vi "试验授权.vi"() -> ()   [LabVIEW 2016]
panel:
  out "簇":T1
  in  "R3加载时间/S  4":dbl=30.0
  in  "R2加载时间/S  4":dbl=30.0
  in  "R1加载时间/S  4":dbl=30.0
  in  "D6加载时间/S  4":dbl=30.0
  in  "D5加载时间/S  4":dbl=30.0
  in  "D4加载时间/S  4":dbl=30.0
  in  "D3加载时间/S 4":dbl=30.0
  in  "D2加载时间/S  4":dbl=30.0
  in  "D1加载时间/S 4":dbl=30.0
  in  "R3加载时间/S  3":dbl=30.0
  in  "R2加载时间/S  3":dbl=30.0
  in  "R1加载时间/S  3":dbl=30.0
  in  "D6加载时间/S  3":dbl=30.0
  in  "D5加载时间/S  3":dbl=30.0
  in  "D4加载时间/S  3":dbl=30.0
  in  "D3加载时间/S 3":dbl=30.0
  in  "D2加载时间/S  3":dbl=30.0
  in  "D1加载时间/S 3":dbl=30.0
  in  "R3加载时间/S  2":dbl=30.0
  in  "R2加载时间/S  2":dbl=30.0
  in  "R1加载时间/S  2":dbl=30.0
  in  "D6加载时间/S  2":dbl=30.0
  in  "D5加载时间/S  2":dbl=30.0
  in  "D4加载时间/S  2":dbl=30.0
  in  "D3加载时间/S 2":dbl=30.0
  in  "D2加载时间/S  2":dbl=30.0
  in  "D1加载时间/S 2":dbl=30.0
  in  "SG18-3百分比":dbl min=0.0 max=100.0 step=1.0
  in  "SG16-3百分比":dbl min=0.0 max=100.0 step=1.0
  in  "SG14百分比":dbl min=0.0 max=100.0 step=1.0
  in  "R3加载时间/S":dbl=30.0
  in  "R2加载时间/S":dbl=30.0
  in  "R1加载时间/S":dbl=30.0
  in  "D6加载时间/S":dbl=30.0
  in  "D5加载时间/S":dbl=30.0
  in  "D4加载时间/S":dbl=30.0
  in  "D3加载时间/S":dbl=30.0
  in  "D2加载时间/S":dbl=30.0
  in  "D1加载时间/S":dbl=30.0
  in  "R3":dbl min=0.0 max=100.0 step=1.0
  in  "R2":dbl min=0.0 max=100.0 step=1.0
  in  "R1":dbl min=0.0 max=100.0 step=1.0
  in  "D6":dbl min=0.0 max=100.0 step=1.0
  in  "D5":dbl min=0.0 max=100.0 step=1.0
  in  "D4":dbl min=0.0 max=100.0 step=1.0
  in  "D3":dbl=30.0 min=0.0 max=100.0 step=1.0
  in  "D2":dbl=50.0 min=0.0 max=100.0 step=1.0
  in  "D1":dbl=50.0 min=0.0 max=100.0 step=1.0
  in  "确定按钮":bool
  # "SG21时间"
  # "SG14时间"
  # "SG16时间"
  # "SG18时间"
  # "百分比"
  # "百分比"
  # "百分比"
  # "百分比"
  # "百分比"
  # "百分比"
  # "百分比"
  # "百分比"
  # "百分比"
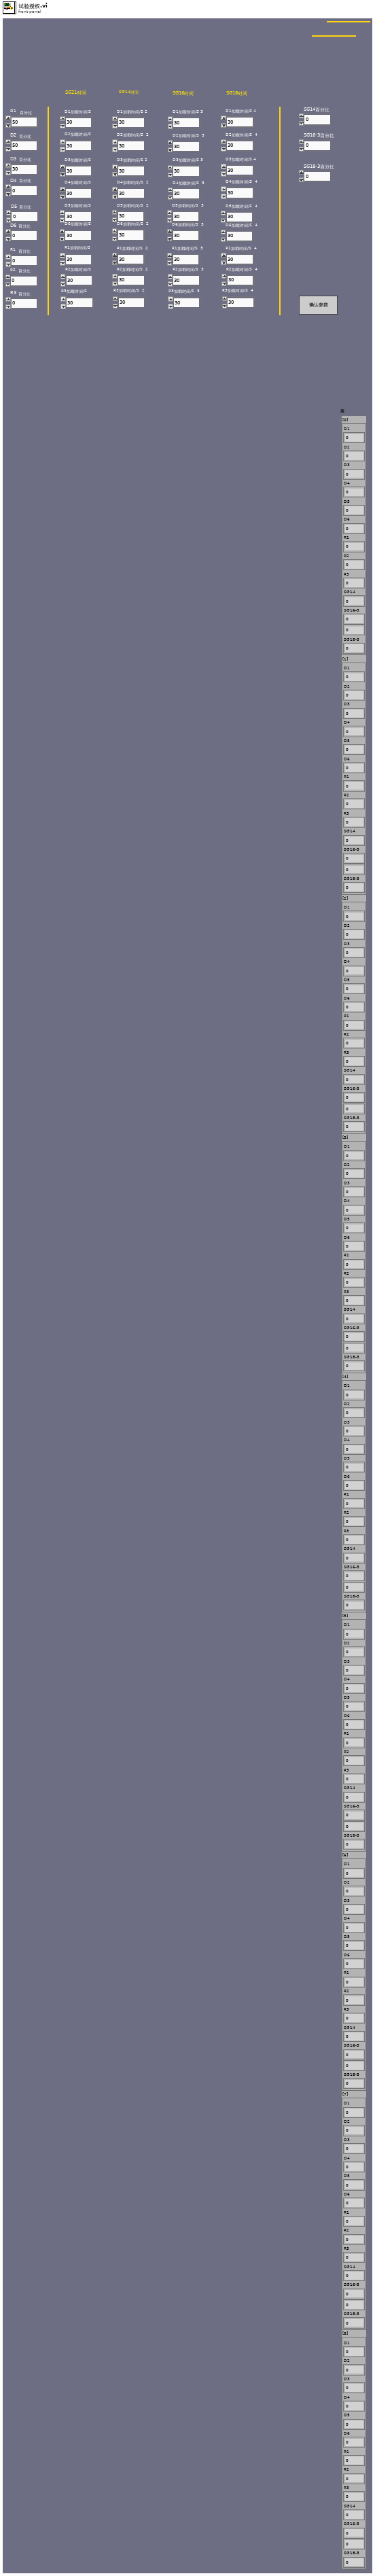
[diagram p1: front panel]
types:
  T1 = cluster{"[0]":cluster{"D1":dbl, "D2":dbl, "D3":dbl, "D4":dbl, "D5":dbl, "D6":dbl, "R1":dbl, "R2":dbl, "R3":dbl, "SG14":dbl, "SG16-3":dbl, dbl, "SG18-3 ":dbl}, "[1]":cluster{"D1":dbl, "D2":dbl, "D3":dbl, "D4":dbl, "D5":dbl, "D6":dbl, "R1":dbl, "R2":dbl, "R3":dbl, "SG14":dbl, "SG16-3":dbl, dbl, "SG18-3 ":dbl}, "[2]":cluster{"D1":dbl, "D2":dbl, "D3":dbl, "D4":dbl, "D5":dbl, "D6":dbl, "R1":dbl, "R2":dbl, "R3":dbl, "SG14":dbl, "SG16-3":dbl, dbl, "SG18-3 ":dbl}, "[3]":cluster{"D1":dbl, "D2":dbl, "D3":dbl, "D4":dbl, "D5":dbl, "D6":dbl, "R1":dbl, "R2":dbl, "R3":dbl, "SG14":dbl, "SG16-3":dbl, dbl, "SG18-3 ":dbl}, "[4]":cluster{"D1":dbl, "D2":dbl, "D3":dbl, "D4":dbl, "D5":dbl, "D6":dbl, "R1":dbl, "R2":dbl, "R3":dbl, "SG14":dbl, "SG16-3":dbl, dbl, "SG18-3 ":dbl}, "[5]":cluster{"D1":dbl, "D2":dbl, "D3":dbl, "D4":dbl, "D5":dbl, "D6":dbl, "R1":dbl, "R2":dbl, "R3":dbl, "SG14":dbl, "SG16-3":dbl, dbl, "SG18-3 ":dbl}, "[6]":cluster{"D1":dbl, "D2":dbl, "D3":dbl, "D4":dbl, "D5":dbl, "D6":dbl, "R1":dbl, "R2":dbl, "R3":dbl, "SG14":dbl, "SG16-3":dbl, dbl, "SG18-3 ":dbl}, "[7]":cluster{"D1":dbl, "D2":dbl, "D3":dbl, "D4":dbl, "D5":dbl, "D6":dbl, "R1":dbl, "R2":dbl, "R3":dbl, "SG14":dbl, "SG16-3":dbl, dbl, "SG18-3 ":dbl}, "[8]":cluster{"D1":dbl, "D2":dbl, "D3":dbl, "D4":dbl, "D5":dbl, "D6":dbl, "R1":dbl, "R2":dbl, "R3":dbl, "SG14":dbl, "SG16-3":dbl, dbl, "SG18-3 ":dbl}}
  T2 = cluster{"D1":dbl, "D2":dbl, "D3":dbl, "D4":dbl, "D5":dbl, "D6":dbl, "R1":dbl, "R2":dbl, "R3":dbl, "SG14":dbl, "SG16-3":dbl, dbl, "SG18-3 ":dbl}
  T3 = cluster{"D1":dbl, "D2":dbl, "D3":dbl, "D4":dbl, "D5":dbl, "D6":dbl, "R1":dbl, "R2":dbl, "R3":dbl, "SG14":dbl, "SG16-3":dbl, dbl, "SG18-3 ":dbl}[]
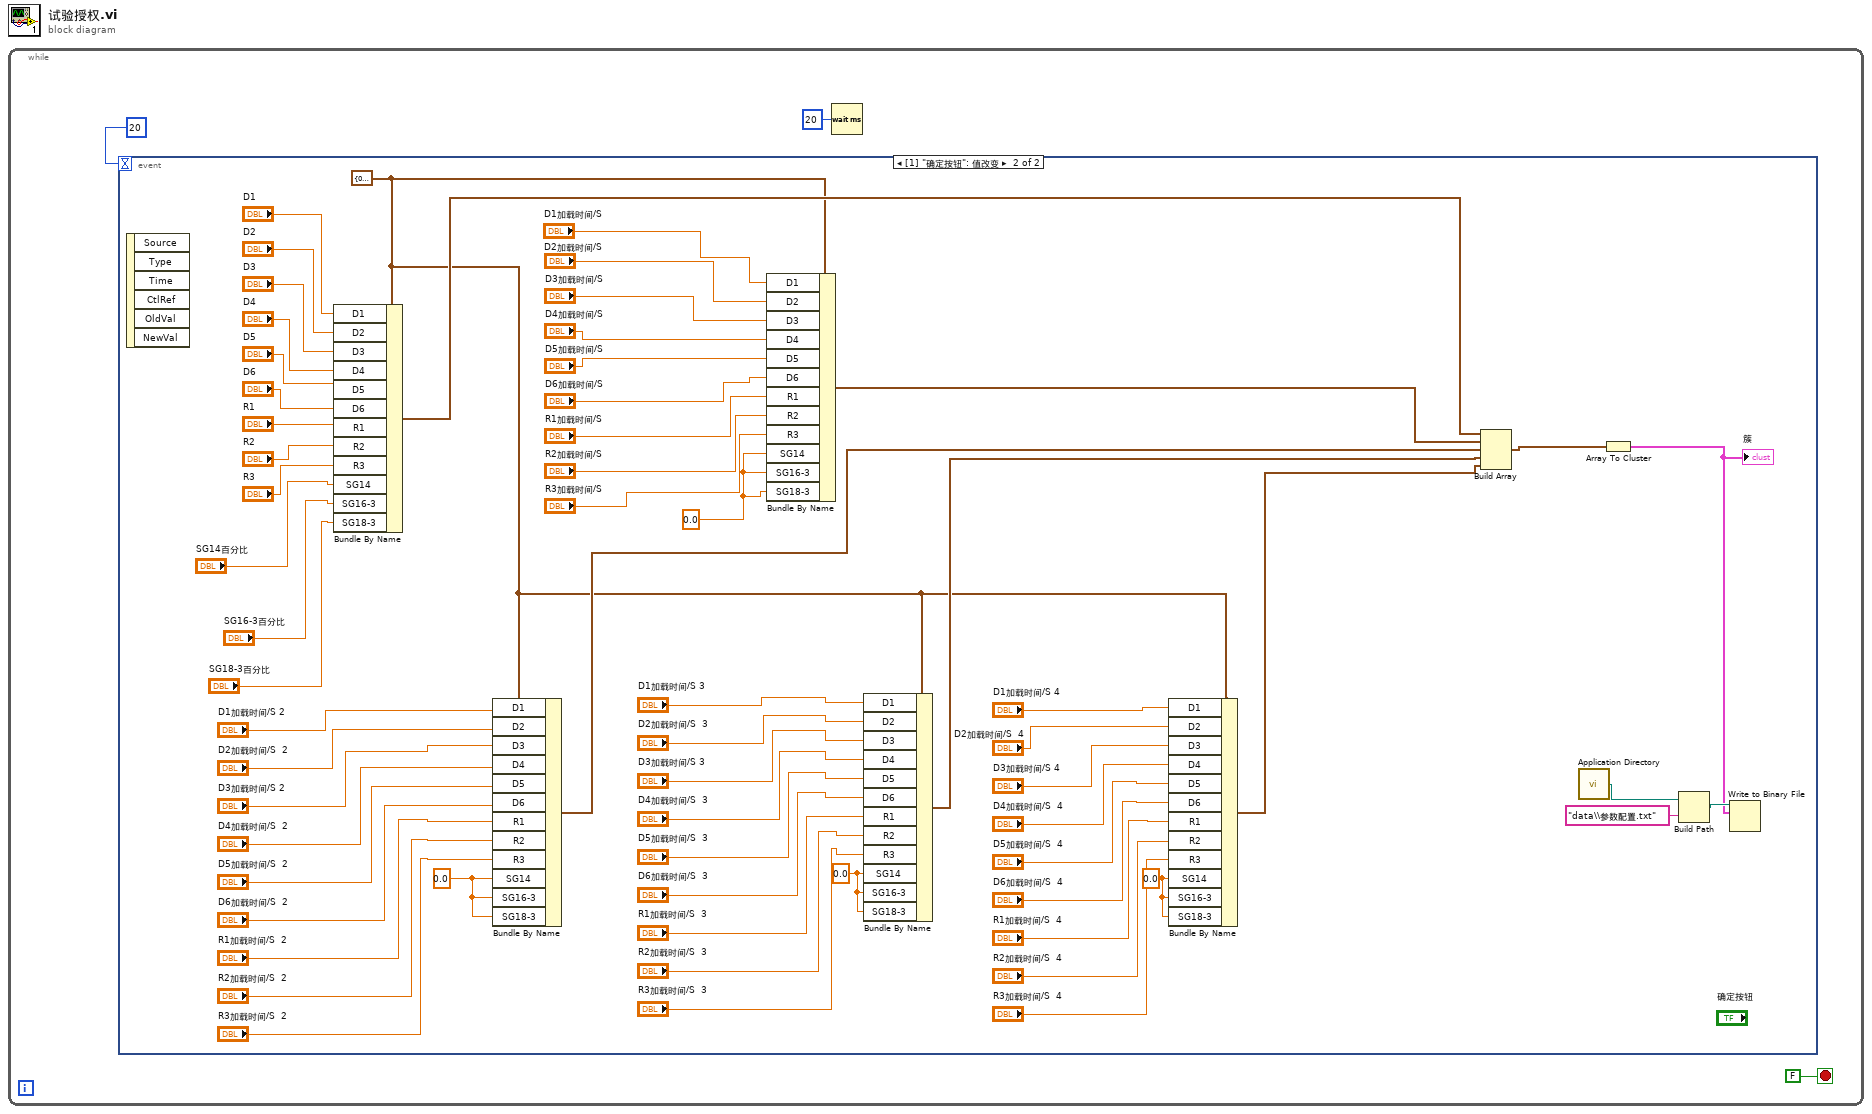
[diagram p0: block diagram]
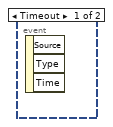
[diagram p2: hidden frame]
diagram:
  n1 = while {
    stop <- FALSE stop-if-true
    n2 = event shown="[1] \"确定按钮\": 值改变" {
      selector: _ -> [_ _]
      dyn-events: _ -> [_ _]
      timeout: 20 -> [_ _]
      event Timeout {
        n3 = event-data() -> ()  [unwired: 1 in, 3 out]
      }
      event "确定按钮": Value Change {
        w6 = 0.0 ("SG14")
        w18 = 0.0 ("SG14")
        w29 = 0.0 ("SG14")
        w39 = 0.0 ("SG14")
        w16 = T2 {"D1"=0.0, "D2"=0.0, "D3"=0.0, "D4"=0.0, "D5"=0.0, "D6"=0.0, "R1"=0.0, "R2"=0.0, "R3"=0.0, "SG14"=0.0, "SG16-3"=0.0, 0.0, "SG18-3 "=0.0}
        n4 = event-data() -> ()  [unwired: 1 in, 6 out]
        n5 = Bundle By Name(cluster=w16, "D1"="D1", "D2"="D2", "D3"="D3", "D4"="D4", "D5"="D5", "D6"="D6", "R1"="R1", "R2"="R2", "R3"="R3", "SG14"="SG14百分比", "SG16-3"="SG16-3百分比", "SG18-3"="SG18-3百分比") -> (w48:T2)
        n6 = Bundle By Name(cluster=w16, "D1"="D1加载时间/S 2", "D2"="D2加载时间/S  2", "D3"="D3加载时间/S 2", "D4"="D4加载时间/S  2", "D5"="D5加载时间/S  2", "D6"="D6加载时间/S  2", "R1"="R1加载时间/S  2", "R2"="R2加载时间/S  2", "R3"="R3加载时间/S  2", "SG14"=w29, "SG16-3"=w29, "SG18-3"=w29) -> (w28:T2)
        n7 = Bundle By Name(cluster=w16, "D1"="D1加载时间/S", "D2"="D2加载时间/S", "D3"="D3加载时间/S", "D4"="D4加载时间/S", "D5"="D5加载时间/S", "D6"="D6加载时间/S", "R1"="R1加载时间/S", "R2"="R2加载时间/S", "R3"="R3加载时间/S", "SG14"=w39, "SG16-3"=w39, "SG18-3"=w39) -> (w47:T2)
        n8 = Bundle By Name(cluster=w16, "D1"="D1加载时间/S 3", "D2"="D2加载时间/S  3", "D3"="D3加载时间/S 3", "D4"="D4加载时间/S  3", "D5"="D5加载时间/S  3", "D6"="D6加载时间/S  3", "R1"="R1加载时间/S  3", "R2"="R2加载时间/S  3", "R3"="R3加载时间/S  3", "SG14"=w18, "SG16-3"=w18, "SG18-3"=w18) -> (w17:T2)
        n9 = Bundle By Name(cluster=w16, "D1"="D1加载时间/S 4", "D2"="D2加载时间/S  4", "D3"="D3加载时间/S 4", "D4"="D4加载时间/S  4", "D5"="D5加载时间/S  4", "D6"="D6加载时间/S  4", "R1"="R1加载时间/S  4", "R2"="R2加载时间/S  4", "R3"="R3加载时间/S  4", "SG14"=w6, "SG16-3"=w6, "SG18-3"=w6) -> (w5:T2)
        n10 = Build Array(w48, w47, w28, w17, w5) -> (w43:T3)
        n11 = call <vilib>:"Application Directory.vi"() -> ("Application Directory"=w46:path)
        n12 = Array To Cluster(array=w43) -> (cluster=w4:T1)
        "簇" <- w4
        n13 = Build Path(base path=w46, name or relative path="data\\参数配置.txt" ("名称或相对路径")) -> (appended path=w44:path)
        n14 = Write to Binary File(file (use dialog)=w44, data=w4) -> ()  [unwired: 4 in, 3 out]
      }
    }
    n15 = Wait (ms)(milliseconds to wait=u32 20 ("等待时间（毫秒）")) -> ()  [unwired: 1 out]
  }
